vi "UDP - Data Channels (SubVI).vi"(6 "test?":bool, 8 "error in":errorcluster, 10 "IP":string, 11 "data in":string) -> (0 "error out":errorcluster, 1 "Channels":T1, 2 "Event":T3 items=["Stop", "Running", "PID", "Up Limit", "Down Limit", "Load Limit"], 3 "Status":T2 items=["Stop", "Ramp Up", "Ramp Down", "Jog Up", "Jog Down", "PID Mode", "PID Ramp"], 4 "Success":bool, 5 "Channels 2":T1)   [LabVIEW 2019]
uses:
  Controls/UDP - Event.ctl
  Controls/UDP - Status.ctl
  Controls/Global - Data UDP.vi
  Controls/Global - IP Address.vi
  Controls/Global - Channel.vi
panel:
  out "unsigned byte array":u8[](array[numeric])
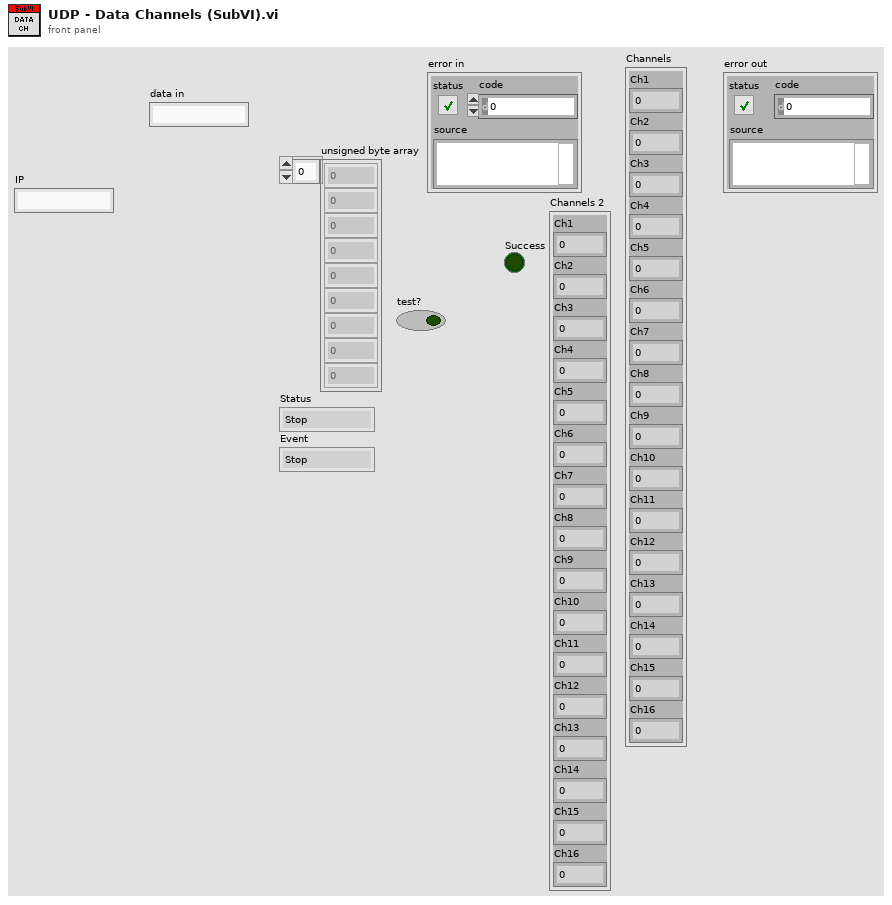
[diagram p1: front panel]
types:
  T1 = cluster{"Ch1":sgl, "Ch2":sgl, "Ch3":sgl, "Ch4":sgl, "Ch5":sgl, "Ch6":sgl, "Ch7":sgl, "Ch8":sgl, "Ch9":sgl, "Ch10":sgl, "Ch11":sgl, "Ch12":sgl, "Ch13":sgl, "Ch14":sgl, "Ch15":sgl, "Ch16":sgl}
  T2 = typedef "UDP - Status.ctl" = u16
  T3 = typedef "UDP - Event.ctl" = u16
  T4 = cluster{"Channels":cluster{"Ch1":sgl, "Ch2":sgl, "Ch3":sgl, "Ch4":sgl, "Ch5":sgl, "Ch6":sgl, "Ch7":sgl, "Ch8":sgl, "Ch9":sgl, "Ch10":sgl, "Ch11":sgl, "Ch12":sgl, "Ch13":sgl, "Ch14":sgl, "Ch15":sgl, "Ch16":sgl}, "Event":T3, "Status":T2, "IP":string}[]
  T5 = cluster{"Channels":cluster{"Ch1":sgl, "Ch2":sgl, "Ch3":sgl, "Ch4":sgl, "Ch5":sgl, "Ch6":sgl, "Ch7":sgl, "Ch8":sgl, "Ch9":sgl, "Ch10":sgl, "Ch11":sgl, "Ch12":sgl, "Ch13":sgl, "Ch14":sgl, "Ch15":sgl, "Ch16":sgl}, "Event":T3, "Status":T2, "IP":string}
  T6 = cluster{"Controller":cluster{"Ch1":sgl, "Ch2":sgl, "Ch3":sgl, "Ch4":sgl, "Ch5":sgl, "Ch6":sgl, "Ch7":sgl, "Ch8":sgl, "Ch9":sgl, "Ch10":sgl, "Ch11":sgl, "Ch12":sgl, "Ch13":sgl, "Ch14":sgl, "Ch15":sgl, "Ch16":sgl}, u8, u8, "IP":string}
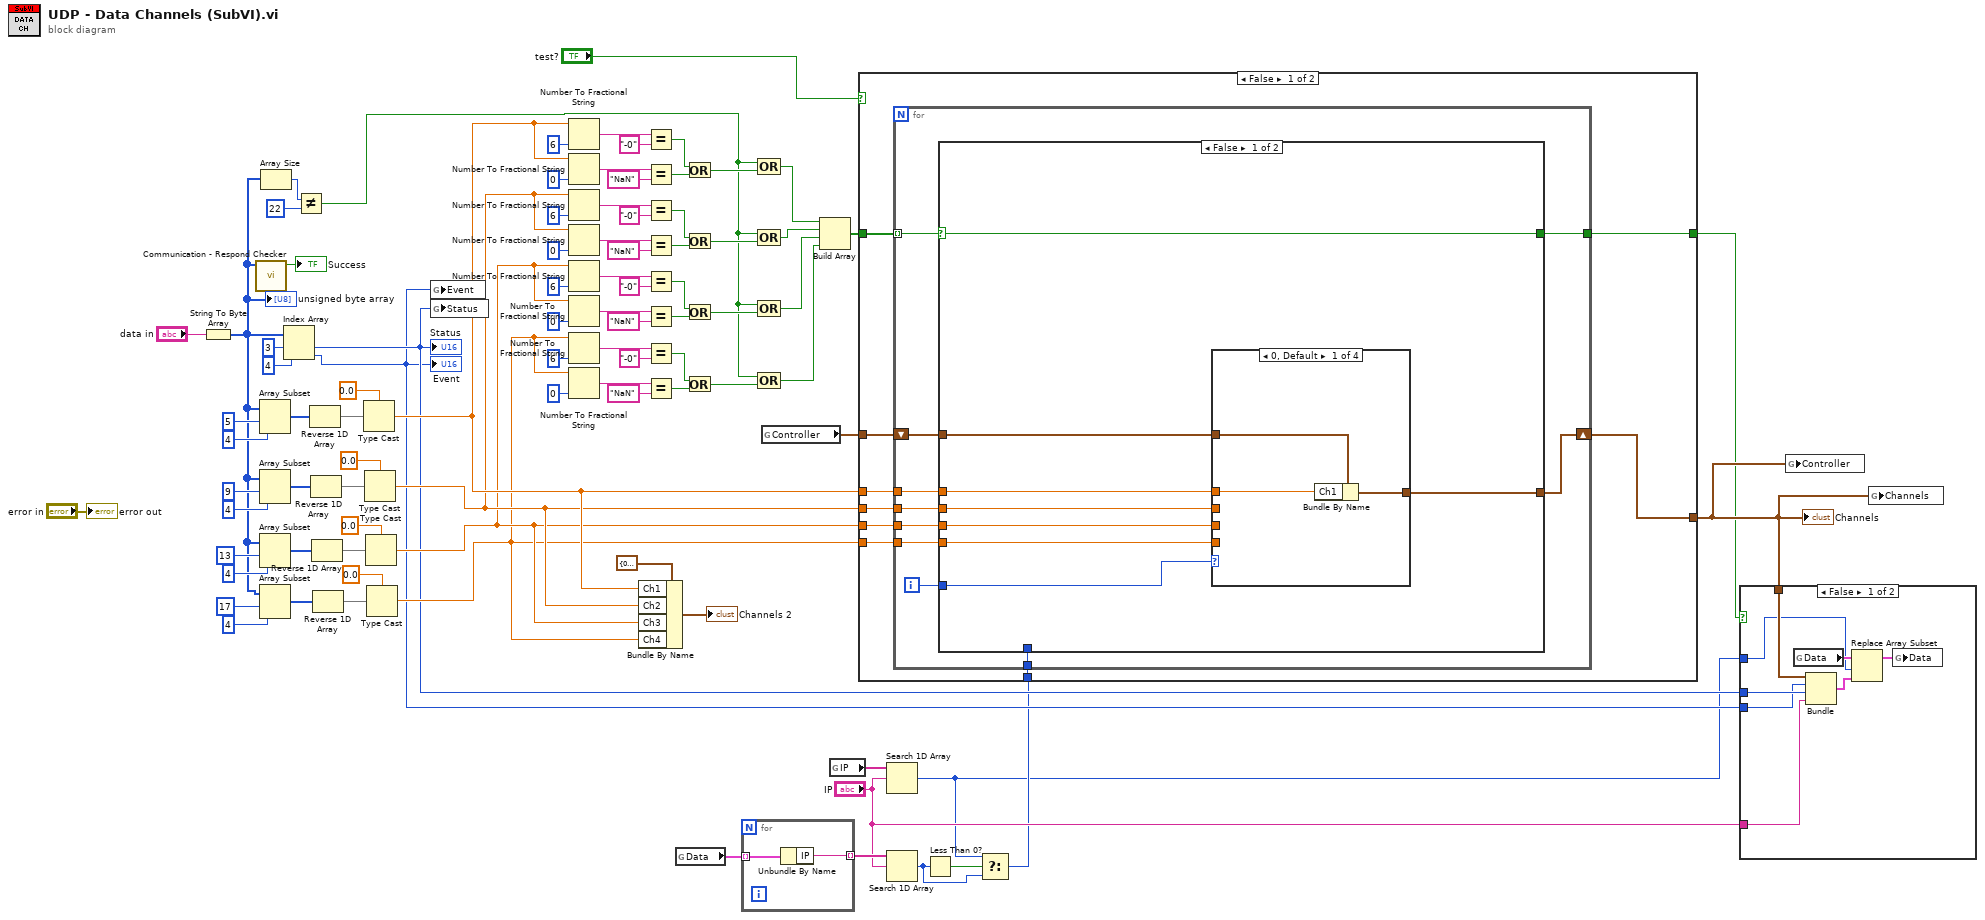
[diagram p0: block diagram]
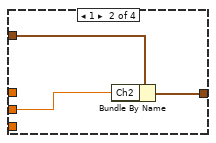
[diagram p3: hidden frame]
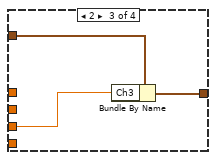
[diagram p4: hidden frame]
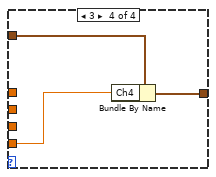
[diagram p5: hidden frame]
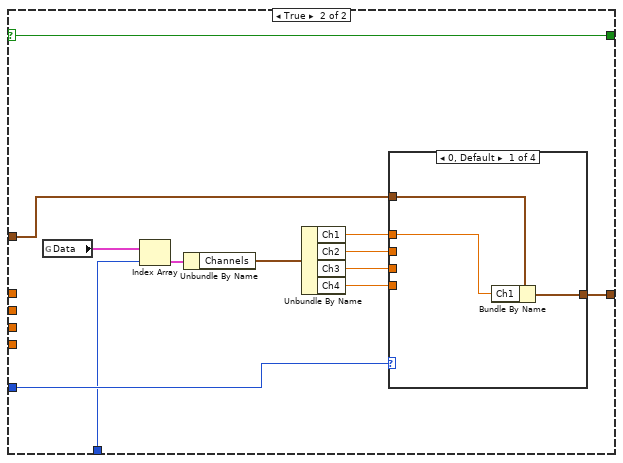
[diagram p6: hidden frame]
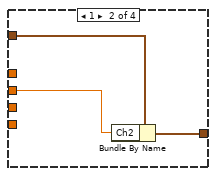
[diagram p7: hidden frame]
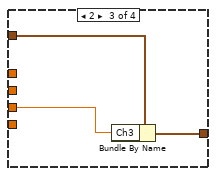
[diagram p8: hidden frame]
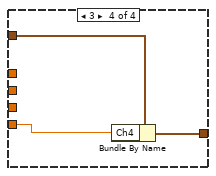
[diagram p9: hidden frame]
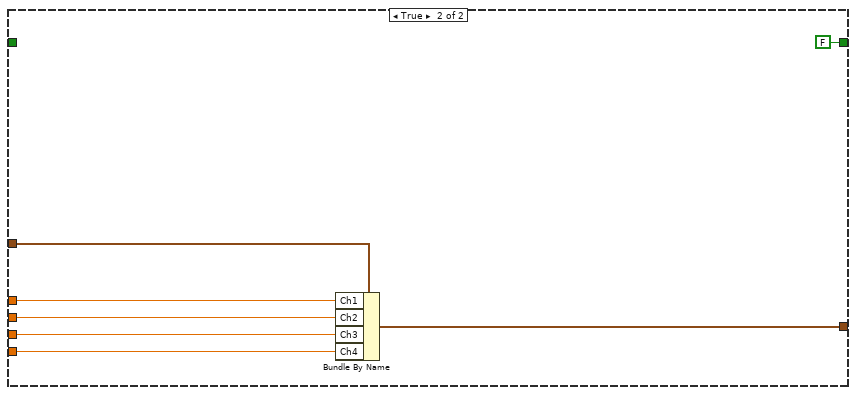
[diagram p10: hidden frame]
diagram:
  n1 = String To Byte Array(string="data in") -> (unsigned byte array=w32:u8[])
  "unsigned byte array" <- w32
  n2 = call "Communication - Respond Checker.vi"("Read Data"=w32) -> ("Success"=→"Success":bool)  [unwired: 10 in]
  n3 = Array Subset(array=w32, index=5, length=4) -> (w72:u8[])
  n4 = Array Subset(array=w32, index=9, length=4) -> (w86:u8[])
  n5 = Array Subset(array=w32, index=13, length=4) -> (w87:u8[])
  n6 = Array Subset(array=w32, index=17, length=4) -> (w88:u8[])
  n7 = Array Size(array=w32) -> (size(s)=w31:i32)
  n8 = Index Array(array=w32, index #1=3 ("index"), index #2=4 ("index")) -> (element #1=w12:u8, element #2=w11:u8)
  "Event" <- w11
  "Status" <- w12
  n9 = Not Equal?(x=w31, y=22) -> (x != y?=w13:bool)
  n10 = Reverse 1D Array(array=w72) -> (reversed array=w73:u8[])
  n11 = Reverse 1D Array(array=w86) -> (reversed array=w80:u8[])
  n12 = Reverse 1D Array(array=w87) -> (reversed array=w83:u8[])
  n13 = Reverse 1D Array(array=w88) -> (reversed array=w84:u8[])
  n14 = Type Cast(type=sgl 0.0, x=w73) -> (*(type *) &x=w29:sgl)
  n15 = Type Cast(type=sgl 0.0, x=w80) -> (*(type *) &x=w28:sgl)
  n16 = Type Cast(type=sgl 0.0, x=w83) -> (*(type *) &x=w27:sgl)
  n17 = Type Cast(type=sgl 0.0, x=w84) -> (*(type *) &x=w26:sgl)
  n18 = global write "Global - Data UDP.vi" "Event"(w11) -> ()
  n19 = global write "Global - Data UDP.vi" "Status"(w12) -> ()
  n20 = Number To Fractional String(number=w29, precision (6)=i16 6) -> (F-format string=w64:string)  [unwired: 2 in]
  n21 = Number To Fractional String(number=w29, precision (6)=i16 0) -> (F-format string=w61:string)  [unwired: 2 in]
  n22 = Number To Fractional String(number=w28, precision (6)=i16 6) -> (F-format string=w51:string)  [unwired: 2 in]
  n23 = Number To Fractional String(number=w28, precision (6)=i16 0) -> (F-format string=w54:string)  [unwired: 2 in]
  n24 = Number To Fractional String(number=w27, precision (6)=i16 6) -> (F-format string=w48:string)  [unwired: 2 in]
  n25 = Number To Fractional String(number=w27, precision (6)=i16 0) -> (F-format string=w45:string)  [unwired: 2 in]
  n26 = Number To Fractional String(number=w26, precision (6)=i16 6) -> (F-format string=w35:string)  [unwired: 2 in]
  n27 = Number To Fractional String(number=w26, precision (6)=i16 0) -> (F-format string=w38:string)  [unwired: 2 in]
  n28 = Bundle By Name(cluster=T1 {"Ch1"=0.0, "Ch2"=0.0, "Ch3"=0.0, "Ch4"=0.0, "Ch5"=0.0, "Ch6"=0.0, "Ch7"=0.0, "Ch8"=0.0, "Ch9"=0.0, "Ch10"=0.0, "Ch11"=0.0, "Ch12"=0.0, "Ch13"=0.0, "Ch14"=0.0, "Ch15"=0.0, "Ch16"=0.0} ("Channels 3"), "Ch1"=w29, "Ch2"=w28, "Ch3"=w27, "Ch4"=w26) -> (→"Channels 2":T1)
  n29 = Equal?(x=w64, y="-0") -> (x = y?=w59:bool)
  n30 = Equal?(x=w61, y="NaN") -> (x = y?=w58:bool)
  n31 = Equal?(x=w51, y="-0") -> (x = y?=w56:bool)
  n32 = Equal?(x=w54, y="NaN") -> (x = y?=w57:bool)
  n33 = Equal?(x=w48, y="-0") -> (x = y?=w43:bool)
  n34 = Equal?(x=w45, y="NaN") -> (x = y?=w42:bool)
  n35 = Equal?(x=w35, y="-0") -> (x = y?=w40:bool)
  n36 = Equal?(x=w38, y="NaN") -> (x = y?=w41:bool)
  n37 = global read "Global - Channel.vi" "Data"() -> (w8:T4)
  n38 = Or(x=w59, y=w58) -> (x .or. y?=w33:bool)
  n39 = Or(x=w56, y=w57) -> (x .or. y?=w20:bool)
  n40 = Or(x=w43, y=w42) -> (x .or. y?=w21:bool)
  n41 = Or(x=w40, y=w41) -> (x .or. y?=w22:bool)
  n42 = for {
    tunnel: w8 -> [w92] mode=indexing
    tunnel: [w91] -> w7 mode=indexing
    n43 = Unbundle By Name(w92) -> ("IP"=w91:string)
  }
  n44 = Compound Arithmetic op=OR(w13, w33) -> (w18:bool)
  n45 = Compound Arithmetic op=OR(w13, w20) -> (w17:bool)
  n46 = Compound Arithmetic op=OR(w13, w21) -> (w16:bool)
  n47 = Compound Arithmetic op=OR(w13, w22) -> (w15:bool)
  n48 = global read "Global - Data UDP.vi" "Controller"() -> (w19:T1)
  n49 = Build Array(w18, w17, w16, w15) -> (w14:bool[])
  n50 = global read "Global - IP Address.vi" "IP"() -> (w9:string[])
  n51 = Search 1D Array(1D array=w9, element="IP") -> (index of element=w2:i32)  [unwired: 1 in]
  n52 = Search 1D Array(1D array=w7, element="IP") -> (index of element=w4:i32)  [unwired: 1 in]
  n53 = Less Than 0?(x=w4) -> (x < 0?=w5:bool)
  n54 = Select(t=w2, s=w5, f=w4) -> (s? t:f=w3:i32)
  n55 = case shown="False" "test?" {
    tunnel: w29 -> [w101 w160]
    tunnel: w28 -> [w100 w159]
    tunnel: w27 -> [w99 w158]
    tunnel: w26 -> [w98 w157]
    tunnel: [w97 w161] -> w10
    tunnel: w19 -> [w95 w162]
    tunnel: w14 -> [w96 _]
    tunnel: w3 -> [w94 _]
    tunnel: [w93 FALSE] -> w1
    frame False {
      n56 = for {
        tunnel: w101 -> [w111]
        tunnel: w100 -> [w110]
        tunnel: w99 -> [w109]
        tunnel: w98 -> [w108]
        shift-right: [w107] -> w97
        shift-left: w95 -> [w106]
        tunnel: w96 -> [w105] mode=indexing
        tunnel: w94 -> [w103]
        tunnel: [w102] -> w93
        i -> [w104]
        n57 = case shown="False" w105 {
          selector: w105 -> [w112 w132]
          tunnel: w111 -> [w119 _]
          tunnel: w110 -> [w115 _]
          tunnel: w109 -> [w114 _]
          tunnel: w108 -> [w113 _]
          tunnel: [w118 w137] -> w107
          tunnel: w106 -> [w117 w143]
          tunnel: w104 -> [w116 w141]
          tunnel: w103 -> [_ w133]
          tunnel: [w112 w132] -> w102
          frame False {
            n58 = case shown="0, Default" w116 {
              tunnel: w119 -> [w122 _ _ _]
              tunnel: [w121 w125 w128 w131] -> w118
              tunnel: w117 -> [w120 w124 w127 w130]
              tunnel: w115 -> [_ w123 _ _]
              tunnel: w114 -> [_ _ w126 _]
              tunnel: w113 -> [_ _ _ w129]
              frame 0, Default {
                n59 = Bundle By Name(cluster=w120, "Ch1"=w122) -> (w121:T1)
              }
              frame 1 {
                n60 = Bundle By Name(cluster=w124, "Ch2"=w123) -> (w125:T1)
              }
              frame 2 {
                n61 = Bundle By Name(cluster=w127, "Ch3"=w126) -> (w128:T1)
              }
              frame 3 {
                n62 = Bundle By Name(cluster=w130, "Ch4"=w129) -> (w131:T1)
              }
            }
          }
          frame True {
            n63 = global read "Global - Channel.vi" "Data"() -> (w136:T4)
            n64 = Index Array(array=w136, index=w133) -> (element=w135:T5)
            n65 = Unbundle By Name(w135) -> ("Channels"=w134:T1)
            n66 = Unbundle By Name(w134) -> ("Ch1"=w142:sgl, "Ch2"=w140:sgl, "Ch3"=w139:sgl, "Ch4"=w138:sgl)
            n67 = case shown="0, Default" w141 {
              tunnel: [w146 w149 w152 w155] -> w137
              tunnel: w143 -> [w145 w148 w151 w154]
              tunnel: w142 -> [w144 _ _ _]
              tunnel: w140 -> [_ w147 _ _]
              tunnel: w139 -> [_ _ w150 _]
              tunnel: w138 -> [_ _ _ w153]
              frame 0, Default {
                n68 = Bundle By Name(cluster=w145, "Ch1"=w144) -> (w146:T1)
              }
              frame 1 {
                n69 = Bundle By Name(cluster=w148, "Ch2"=w147) -> (w149:T1)
              }
              frame 2 {
                n70 = Bundle By Name(cluster=w151, "Ch3"=w150) -> (w152:T1)
              }
              frame 3 {
                n71 = Bundle By Name(cluster=w154, "Ch4"=w153) -> (w155:T1)
              }
            }
          }
        }
      }
    }
    frame True {
      n72 = Bundle By Name(cluster=w162, "Ch1"=w160, "Ch2"=w159, "Ch3"=w158, "Ch4"=w157) -> (w161:T1)
    }
  }
  "Channels" <- w10
  n73 = case shown="False" w1 {
    tunnel: w12 -> [w167 _]
    tunnel: w11 -> [w166 _]
    tunnel: w10 -> [w165 _]
    tunnel: "IP" -> [w164 _]
    tunnel: w2 -> [w163 _]
    frame False {
      n74 = global read "Global - Channel.vi" "Data"() -> (w170:T4)
      n75 = Bundle("Controller"=w165, w166, w167, "IP"=w164) -> (w169:T6)  [unwired: 1 in]
      n76 = Replace Array Subset(array=w170, new element=w169, index=w163) -> (w168:T4)
      n77 = global write "Global - Channel.vi" "Data"(w168) -> ()
    }
    frame True {
    }
  }
  n78 = global write "Global - Data UDP.vi" "Controller"(w10) -> ()
  n79 = global write "Global - Data UDP.vi" "Channels"(w10) -> ()
  "error out" <- "error in"
